vi "Check-Create Default Data Path.vi"(8 "error in":errorcluster) -> (0 "error out":errorcluster, 3 "Default Data Path":path)   [LabVIEW 2011]
doc: "Creates the default data path if it doesn't exist.\n\n\nVersion 1.0 - 02/13/2013\n\nPhaeron, Inc.\nwww.phaeron.com\ninfo@phaeron.com"
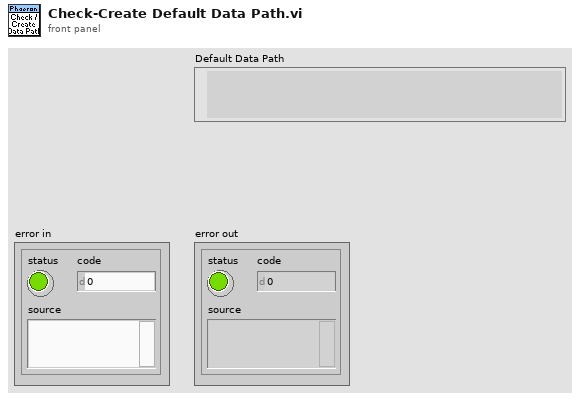
[diagram p1: front panel]
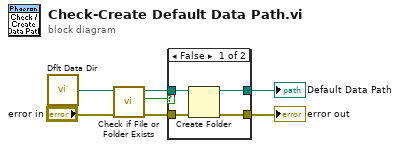
[diagram p0: block diagram]
diagram:
  n1 = call <vilib>:"Dflt Data Dir.vi"() -> ("App:Default Data Directory"=w2:path)
  n2 = call <vilib>:"Check if File or Folder Exists.vi"("error in (no error)"="error in", "path"=w2) -> ("error out"=w6:errorcluster, "file or folder exists?"=w4:bool, "dup path"=w5:path)  [unwired: 7 in]
  n3 = case shown="False" w4 {
    tunnel: [w11 w13] -> w1
    tunnel: [w10 w12] -> w3
    tunnel: w6 -> [w9 w12]
    tunnel: w5 -> [w8 w13]
    frame False {
      n4 = Create Folder(path (use dialog)=w8, error in=w9) -> (created path=w11:path, error out=w10:errorcluster)  [unwired: 1 in, 1 out]
    }
    frame True {
    }
  }
  "Default Data Path" <- w1
  "error out" <- w3
